vi "ScanAEGroup.vi"(8 "error in (no error)":errorcluster, 11 "AE Group String":string) -> (0 "error out":errorcluster, 3 "AE Group":T1(ring))   [LabVIEW 2017, in "Client.lvlib" / "ParserSorter.lvlib"]
uses:
  ParserSorter.lvlib
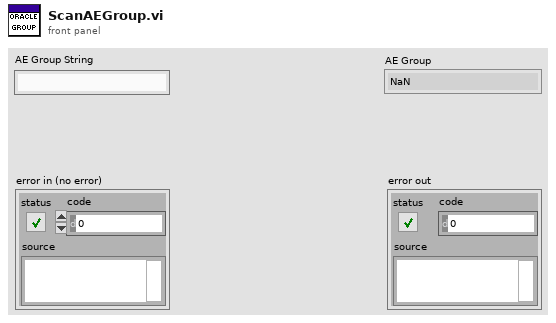
[diagram p1: front panel]
types:
  T1 = enum32{"NaN", "AE-Germany", "AE-Poland", "AE-Switzerland", "AE-Czech Republic", "AE-Hungary", "AE-Romania", "AE-Slovakia", "AE-Slovenia"}
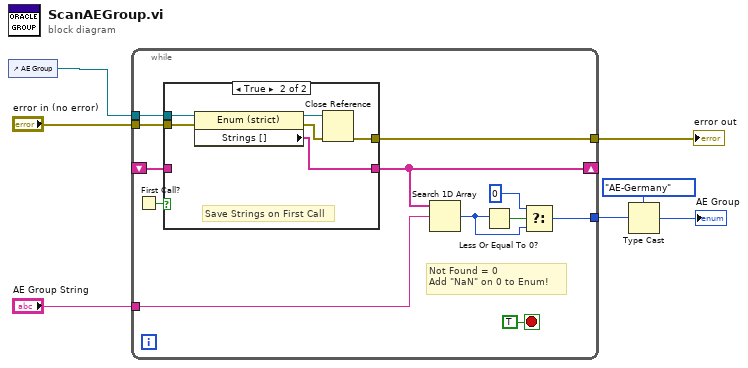
[diagram p0: block diagram]
diagram:
  n1 = control-ref of="AE Group"() -> (w1:refnum<vi>)
  n2 = while {
    tunnel: w1 -> [w19]
    shift-right: [w13] -> _
    shift-left: _ -> [w16]
    tunnel: [w15] -> w6
    tunnel: "error in (no error)" -> [w14]
    tunnel: [w9] -> w4
    tunnel: "AE Group String" -> [w8]
    stop <- TRUE stop-if-true
    # "Not Found = 0\nAdd \"NaN\" on 0 to Enum!"
    n3 = First Call?() -> (First Call?: T/F=w18:bool)
    n4 = case shown="True" w18 {
      tunnel: w19 -> [_ w27]
      tunnel: [w21 w25] -> w13
      tunnel: w16 -> [w21 _]
      tunnel: [w20 w23] -> w15
      tunnel: w14 -> [w20 w22]
      frame False {
      }
      frame True {
        # "Save Strings on First Call"
        n5 = property class="Enum (strict)"(reference=w27, error in=w22) -> (reference out=w26:refnum<vi>, error out=w24:errorcluster, "Strings []"=w25:string[])
        n6 = Close Reference(reference=w26, error in (no error)=w24) -> (error out=w23:errorcluster)
      }
    }
    n7 = Search 1D Array(1D array=w13, element=w8) -> (index of element=w10:i32)  [unwired: 1 in]
    n8 = Less Or Equal To 0?(x=w10) -> (x <= 0?=w12:bool)
    n9 = Select(t=0 ("Enum Index"), s=w12, f=w10) -> (s? t:f=w9:i32)
  }
  "error out" <- w6
  n10 = Type Cast(type=T1."AE-Germany" ("AE Group"), x=w4) -> (*(type *) &x=→"AE Group":T1)
